vi "DAQ Relay States - Update.vi"(0 "TSM Context":T3, 5 "DAQ States - Out":T1[](array[typedef]) {"Relay Action" items=["Open Relay"=20, "Close Relay"=21]}, 11 "error in (no error)":errorcluster) -> (15 "error out":errorcluster)   [LabVIEW 2019]
uses:
  <vilib>/NI_TestStand_SemiconductorModule/NI_TestStand_Semiconductor_Module.lvlibp/PinMap/General/SemiconductorModuleContext.ctl
  typedefs/DAQ Relay Pins.ctl
  <vilib>/NI_TestStand_SemiconductorModule/NI_TestStand_Semiconductor_Module.lvlibp/1abvi3w/instr.lib/niSwitch/niswitch.llb/niSwitch Relay Action.ctl
  TSM Context Data Access/Public/Properties/DAQ Relay States - Write.vi
  TSM Context Data Access/TSM Context Data Access.lvclass
  <vilib>/NI_TestStand_SemiconductorModule/NI_TestStand_Semiconductor_Module.lvlibp
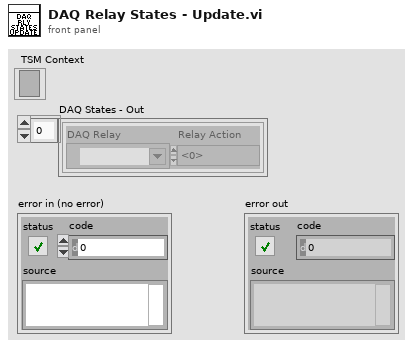
[diagram p1: front panel]
types:
  T1 = typedef "DAQ Relay Pins.ctl" = cluster{"DAQ Relay":tag, "Relay Action":T2}
  T2 = typedef "NI_TestStand_Semiconductor_Module.lvlibp/niSwitch Relay Action.ctl" = i32
  T3 = typedef "NI_TestStand_Semiconductor_Module.lvlibp/SemiconductorModuleContext.ctl" = refnum<k7>
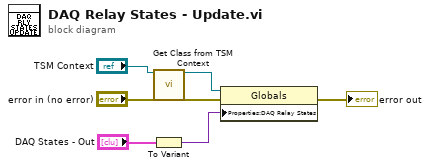
[diagram p0: block diagram]
diagram:
  n1 = call "Get Class from TSM Context.vi"("TSM Context"="TSM Context") -> ("Global Memory Class"=w6:refnum<class "TSM Context Data Access.lvclass">)  [unwired: 14 in]
  n2 = To Variant(anything="DAQ States - Out") -> (Variant=w5:variant)
  n3 = property class="Globals"(reference=w6, error in="error in (no error)", "Properties:DAQ Relay States"=w5) -> (error out=→"error out":errorcluster)  [unwired: 1 out]
